vi "SwerveMath.vi"(0 "Strafe Joystick Axes":cluster{"X":dbl, "Y":dbl}, 1 "Trigger Axes":cluster{"Left":dbl, "Right":dbl}, 2 "Center of Rotation Joystick":cluster{"Left":dbl, "Right":dbl}, 5 "FieldCentric? (T)":bool=TRUE, 7 "Angle (degrees; 0 = right)":dbl, 9 "Strafe Multiplier":dbl, 11 "Rotation Multiplier":dbl) -> (6 "Motor Speeds":dbl[](array[numeric]), 10 "Motor Angles":dbl[](array[numeric]))   [LabVIEW 2014, in "Team900SwerveDrive.lvlib"]
uses:
  Team900SwerveDrive.lvlib
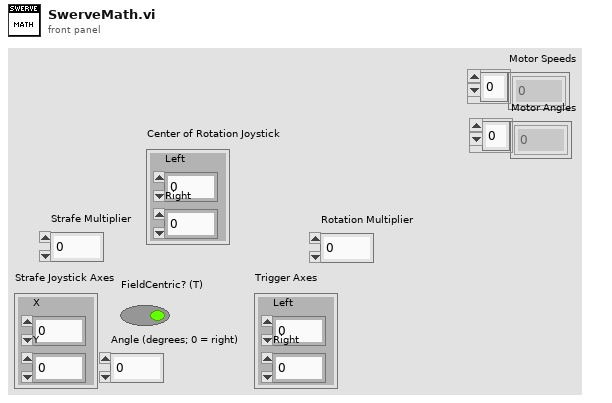
[diagram p1: front panel]
types:
  T1 = cluster{"normalized array[0]":dbl, "normalized array[1]":dbl, "normalized array[2]":dbl, "normalized array[3]":dbl}
  T2 = cluster{"FL Angle":dbl, "FR Angle":dbl, "RL Angle":dbl, "RR Angle":dbl}
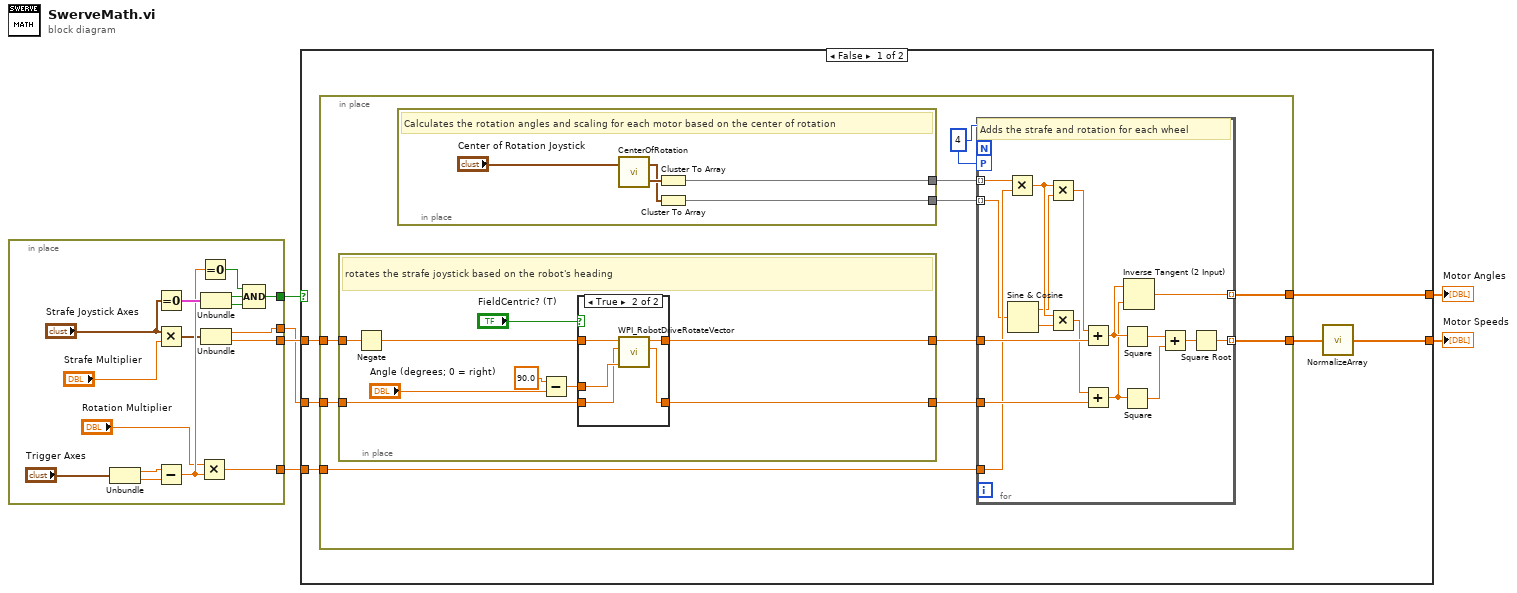
[diagram p0: block diagram]
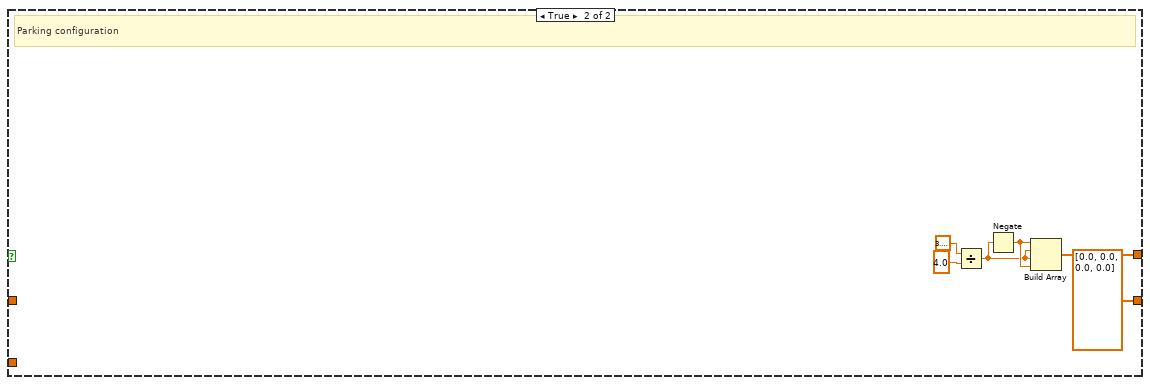
[diagram p3: hidden frame]
diagram:
  n1 = in-place {
    in-place-border: [w15] -> w6
    in-place-border: [w14] -> w5
    in-place-border: [w13] -> w4
    in-place-border: [w11] -> w3
    n2 = Unbundle("Trigger Axes") -> ("Left"=w18:dbl, "Right"=w19:dbl)
    n3 = Equal To 0?(x="Strafe Joystick Axes") -> (x = 0?=w21:cluster{"X":bool, "Y":bool})
    n4 = Multiply(x="Strafe Joystick Axes", y="Strafe Multiplier") -> (x*y=w9:cluster{"X":dbl, "Y":dbl})
    n5 = Subtract(x=w18, y=w19) -> (x-y=w12:dbl)
    n6 = Multiply(x="Rotation Multiplier", y=w12) -> (x*y=w11:dbl)
    n7 = Equal To 0?(x=w12) -> (x = 0?=w7:bool)
    n8 = Unbundle(w21) -> ("X"=w17:bool, "Y"=w16:bool)
    n9 = Unbundle(w9) -> ("X"=w13:dbl, "Y"=w14:dbl)
    n10 = Compound Arithmetic op=AND(w7, w17, w16) -> (w15:bool)
  }
  n11 = case shown="False" w6 {
    tunnel: [w25 w82] -> w1
    tunnel: [w23 dbl[] [0.0, 0.0, 0.0, 0.0] ("appended array")] -> w2
    tunnel: w5 -> [w28 _]
    tunnel: w4 -> [w27 _]
    tunnel: w3 -> [w26 _]
    frame False {
      n12 = in-place {
        in-place-border: [w36] -> w24
        in-place-border: [w35] -> w25
        in-place-border: w28 -> [w33]
        in-place-border: w27 -> [w32]
        in-place-border: w26 -> [w31]
        w34 = 4
        n13 = in-place {
          in-place-border: [w52] -> w38
          in-place-border: [w51] -> w37
          in-place-border: w33 -> [w47]
          in-place-border: w32 -> [w46]
          # "rotates the strafe joystick based on the robot's heading"
          n14 = Negate(x=w47) -> (-x=w48:dbl)
          n15 = Subtract(x=90.0 ("y"), y="Angle (degrees; 0 = right)") -> (x-y=w49:dbl)
          n16 = case shown="True" "FieldCentric? (T)" {
            tunnel: w48 -> [w54 w59]
            tunnel: [w54 w58] -> w52
            tunnel: [w53 w57] -> w51
            tunnel: w49 -> [_ w56]
            tunnel: w46 -> [w53 w55]
            frame False {
            }
            frame True {
              n17 = call <vilib>:"WPI_RobotDriveRotateVector.vi"("Angle"=w56, "X"=w55, "Y"=w59) -> ("X'"=w57:dbl, "Y'"=w58:dbl)  [unwired: 7 out]
            }
          }
        }
        n18 = in-place {
          in-place-border: [w40] -> w30
          in-place-border: [w41] -> w29
          # "Calculates the rotation angles and scaling for each motor based on the center of rotation"
          n19 = call "CenterOfRotation.vi"("Center of Rotation Joystick Axes"="Center of Rotation Joystick") -> ("Rotation Multipliers"=w43:T1, "Rotation Angle Cluster"=w42:T2)  [unwired: 1 in]
          n20 = Cluster To Array(cluster=w43) -> (array=w40:dbl[])
          n21 = Cluster To Array(cluster=w42) -> (array=w41:dbl[])
        }
        n22 = for {
          N: w34 -> [_]
          tunnel: w38 -> [w76]
          tunnel: w37 -> [w75]
          tunnel: w31 -> [w74]
          tunnel: [w73] -> w36 mode=indexing
          tunnel: [w72] -> w35 mode=indexing
          workers-P: w34 -> [_]
          tunnel: w30 -> [w61] mode=indexing
          tunnel: w29 -> [w60] mode=indexing
          # "Adds the strafe and rotation for each wheel"
          n23 = Multiply(x=w61, y=w74) -> (x*y=w64:dbl)
          n24 = Sine & Cosine(0:w60) -> (1:w63:dbl, 2:w62:dbl)
          n25 = Multiply(x=w64, y=w63) -> (x*y=w67:dbl)
          n26 = Multiply(x=w64, y=w62) -> (x*y=w68:dbl)
          n27 = Add(x=w67, y=w76) -> (x+y=w66:dbl)
          n28 = Add(x=w68, y=w75) -> (x+y=w65:dbl)
          n29 = Square(x=w66) -> (x^2=w70:dbl)
          n30 = Square(x=w65) -> (x^2=w69:dbl)
          n31 = Inverse Tangent (2 Input)(1:w65, 2:w66) -> (0:w72:dbl)
          n32 = Add(x=w70, y=w69) -> (x+y=w71:dbl)
          n33 = Square Root(x=w71) -> (sqrt(x)=w73:dbl)
        }
      }
      n34 = call "NormalizeArray.vi"("array"=w24) -> ("normalized array"=w23:dbl[])
    }
    frame True {
      # "Parking configuration"
      n35 = Divide(x=3.141592653589793, y=4.0) -> (x/y=w79:dbl)
      n36 = Negate(x=w79) -> (-x=w80:dbl)
      n37 = Build Array(w80, w79, w79, w80) -> (w82:dbl[])
    }
  }
  "Motor Speeds" <- w2
  "Motor Angles" <- w1
